vi "RSZVB Trace Response Single Sweep Data Forward.vi"(8 "error in (no error)":errorcluster {"code" format="%.0x"}, 9 "Sweep Number (1)":i32=1, 10 "Channel (Trace) (1)":i32=1, 11 "VISA session":refnum<visa-resource-name>) -> (0 "error out":errorcluster {"code" format="%.0x"}, 2 "Trace Data":dbl[](array[numeric]) format="%^.3e", 3 "dup VISA session":refnum<visa-resource-name>)   [LabVIEW 2011]
doc: "This VI reads the response values of a trace acquired in single sweep mode (INITiate<Ch>:CONTinuous OFF).\n\nRemote-control command(s):\nFORMat[:DATA] REAL ,32\nCALCulate<Ch/Tr>:DATA:NSWeep:FIRSt? SDATa,<Forward_Count>"
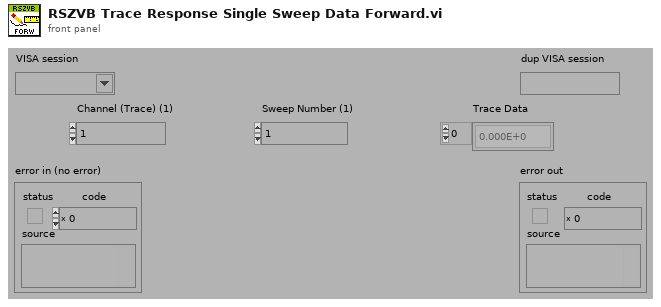
[diagram p1: front panel]
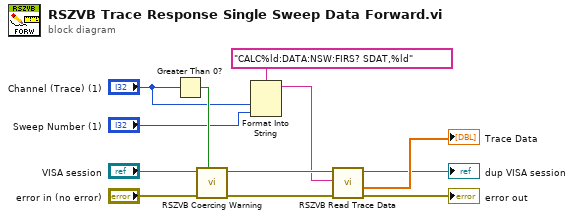
[diagram p0: block diagram]
diagram:
  n1 = Greater Than 0?(x="Channel (Trace) (1)") -> (x > 0?=w8:bool)
  n2 = call "RSZVB Coercing Warning.vi"("In Range?"=w8, "error in (no error)"="error in (no error)", "VISA session"="VISA session") -> ("error out"=w11:errorcluster, "dup VISA session"=w10:refnum<visa-resource-name>)  [unwired: 7 in]
  n3 = Format Into String(format string="CALC%ld:DATA:NSW:FIRS? SDAT,%ld", "Channel (Trace) (1)", "Sweep Number (1)") -> (resulting string=w9:string)  [unwired: 2 in, 1 out]
  n4 = call "RSZVB Read Trace Data.vi"("error in (no error)"=w11, "Buffer"=w9, "VISA session"=w10) -> ("error out"=→"error out":errorcluster, "Trace Data"=→"Trace Data":dbl[], "dup VISA session"=→"dup VISA session":refnum<visa-resource-name>)  [unwired: 6 in]
